vi "Update uService List.vi"(8 "error in (no error)":errorcluster, 10 "All uS?":bool, 11 "Common GUI v3 in":refnum<class "Common GUI v3.lvclass">) -> (0 "error out":errorcluster, 1 "Check currently displayed":set{string}(c389), 2 "For ComboBox":cluster{"ID":string, "ID":string}[](array[cluster]), 3 "Map":map{string, cluster{bool, "Last Pat":timestamp}}(c390), 5 "Common GUI v3 out":refnum<class "Common GUI v3.lvclass">)   [LabVIEW 2026, in "TALOS.lvlib" / "Common GUI v3.lvlib" / "Common GUI v3.lvclass"]
uses:
  Common GUI v3.lvclass
  Classes/uService List/uService List.lvclass/uService List.ctl
  Ancestor/Ancestor/Ancestor.lvclass/Ancestor.ctl
  Classes/uService List/Get all IDs.vi
  Classes/uService List/Get Properties.vi
  Support VIs/Generate Error.vi
  FGV/Error Memory/Get Error Description.vi
  Support VIs/Get PC name.vi
  Ancestor/Ancestor/Read ID.vi
  Support VIs/Get Class Name.vi
  <vilib>/Utility/error.llb/Clear Errors.vi
  FGV/Error Memory/Error Memory Core.vi
  <vilib>/AdvancedString/Delimited String to 1D String Array.vi
  <vilib>/AdvancedString/Delimited String to 1D String Array (string).vi
  Support VIs/Circus Root Path.vi
  FGV/Error Memory/Error Crt Lvl checker.vi
  FGV/Error Memory/Error Memory Core.vi/40c8088d-b597-4017-91af-faa98e00292e.vi
  FGV/Error Memory/Error Memory Core.vi/d4a3ab98-063c-4e44-b43d-fbdcfe6c2be2.vi
  Support VIs/Global Memory.vi
  <vilib>/Utility/LVClass/Get LV Class Name.vi
  Support VIs/Is in Packed Library.vi
  Support VIs/TALOS Root path.vi
  Support VIs/Read CSV worksheet.vi
  Support VIs/Global Constants.vi
  <vilib>/Utility/error.llb/General Error Handler.vi
  builds/Actor Framework PPL/Actor Framework.lvlibp/1abvi3w/vi.lib/ActorFramework/Message Enqueuer/Message Enqueuer.lvclass
  Ancestor/Ancestor/Ancestor.lvclass
  <vilib>/Comparison/Equal/Equal Functor/Equal Functor.lvclass
  Classes/uService List/uService List.lvclass
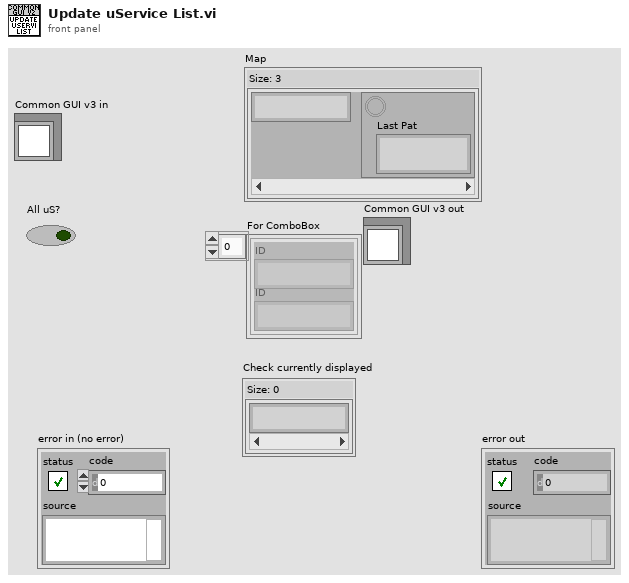
[diagram p1: front panel]
types:
  T1 = typedef "TALOS.lvlib/Classes.lvlib/uService List.lvclass/uService Properties.ctl" = cluster{"uService Queue":refnum<class "Message Enqueuer.lvclass">, "Last Pat":timestamp, "Online":bool, "Vi Ref":refnum<vi>, "Class name":string, "GUI":bool, "FP Items Refs Map":map{string, refnum<vi>}, "Remote GUI":bool, "Remote Window":refnum<vi>}
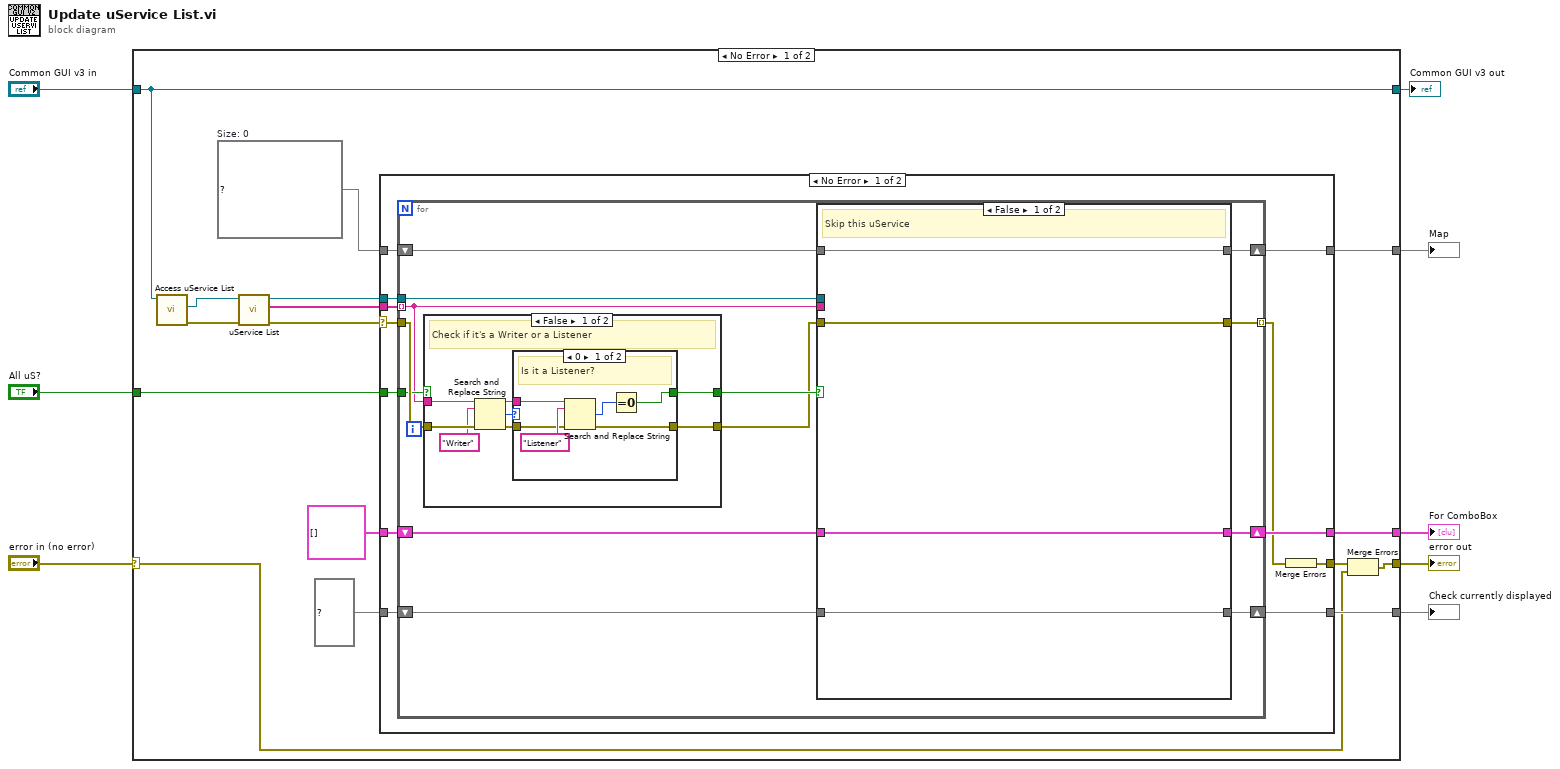
[diagram p0: block diagram]
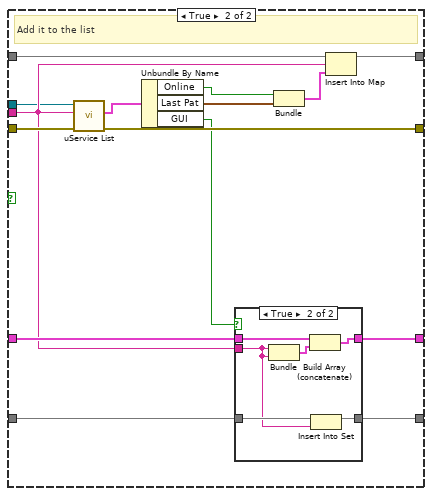
[diagram p2: hidden frame]
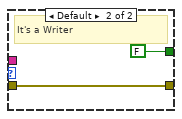
[diagram p4: hidden frame]
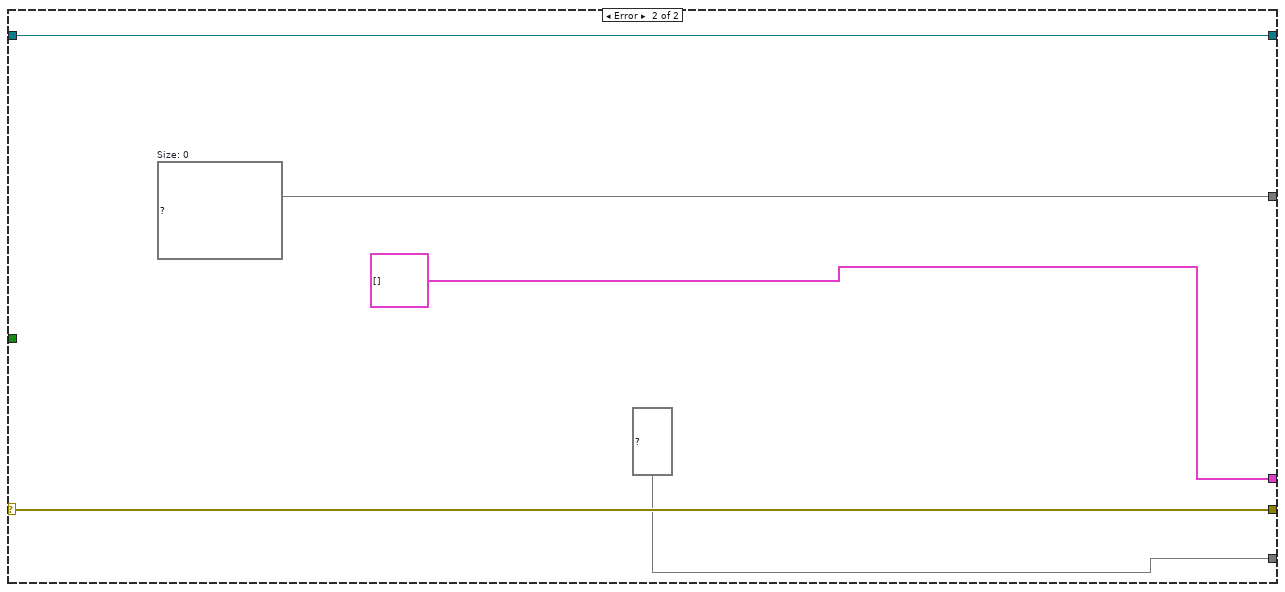
[diagram p7: hidden frame]
diagram:
  n1 = case shown="No Error" "error in (no error)" {
    selector: "error in (no error)" -> [w15 w103]
    tunnel: [w16 w103] -> w7
    tunnel: [w23 w102] -> w6
    tunnel: [w22 cluster{"ID":string, "ID":string}[] []] -> w5
    tunnel: [w17 set{string} {} ("Check currently displayed")] -> w4
    tunnel: "Common GUI v3 in" -> [w12 w99]
    tunnel: [w12 w99] -> w2
    tunnel: "All uS?" -> [w9 _]
    frame No Error {
      w24 = map{string, cluster{bool, "Last Pat":timestamp}} {}  # Size: 0
      n2 = call-dynamic "Access uService List.vi"("Ancestor in"=w12) -> ("error out"=w14:errorcluster, "uService List out"=w13:refnum<class "uService List.lvclass">)  [unwired: 8 in, 1 out]
      n3 = call-poly "uService List.vi"("error in (no error)"=w14, "uService List"=w13) -> ("error out"=w21:errorcluster, "All IDs"=w11:string[], "uService List out"=w10:refnum<class "uService List.lvclass">)  [unwired: 7 in]
      n4 = case shown="No Error" w21 {
        selector: w21 -> [w32 w95]
        tunnel: w24 -> [w36 w98]
        tunnel: [w35 w98] -> w23
        tunnel: [w34 w97] -> w22
        tunnel: w11 -> [w33 _]
        tunnel: cluster{"ID":string, "ID":string}[] [] -> [w31 w97]
        tunnel: [w29 w95] -> w19
        tunnel: set{string} {} ("Check currently displayed") -> [w28 w96]
        tunnel: [w27 w96] -> w17
        tunnel: w10 -> [w26 _]
        tunnel: w9 -> [w25 _]
        frame No Error {
          n5 = for {
            tunnel: w33 -> [w39] mode=indexing
            tunnel: w32 -> [w49]
            shift-right: [w48] -> w35
            shift-left: w36 -> [w47]
            shift-right: [w45] -> w34
            shift-left: w31 -> [w46]
            tunnel: [w44] -> w30 mode=indexing
            shift-right: [w42] -> w27
            shift-left: w28 -> [w43]
            tunnel: w26 -> [w41]
            tunnel: w25 -> [w40]
            n6 = case shown="False" w40 {
              selector: w40 -> [_ w94]
              tunnel: w39 -> [w84 _]
              tunnel: [w77 w94] -> w38
              tunnel: w49 -> [w83 w93]
              tunnel: [w78 w93] -> w37
              frame False {
                # "Check if it's a Writer or a Listener"
                n7 = Search and Replace String(input string=w84, search string="Writer", error in=w83) -> (result string=w79:string, number of replacements=w80:i32, error out=w81:errorcluster)  [unwired: 5 in, 1 out]
                n8 = case shown="0" w80 {
                  tunnel: w81 -> [w88 w92]
                  tunnel: w79 -> [w89 _]
                  tunnel: [w87 w92] -> w78
                  tunnel: [w85 FALSE] -> w77
                  frame 0 {
                    # "Is it a Listener?"
                    n9 = Search and Replace String(input string=w89, search string="Listener", error in=w88) -> (number of replacements=w86:i32, error out=w87:errorcluster)  [unwired: 5 in, 2 out]
                    n10 = Equal To 0?(x=w86) -> (x = 0?=w85:bool)
                  }
                  frame Default {
                    # "It's a Writer"
                  }
                }
              }
              frame True {
                # "Parse all uS"
              }
            }
            n11 = case shown="False" w38 {
              tunnel: [w53 w68] -> w48
              tunnel: w47 -> [w53 w67]
              tunnel: w46 -> [w51 w66]
              tunnel: [w51 w65] -> w45
              tunnel: w37 -> [w52 w64]
              tunnel: [w52 w63] -> w44
              tunnel: w43 -> [w50 w58]
              tunnel: [w50 w57] -> w42
              tunnel: w39 -> [_ w56]
              tunnel: w41 -> [_ w54]
              frame False {
                # "Skip this uService"
              }
              frame True {
                # "Add it to the list"
                n12 = call-poly "uService List.vi"("error in (no error)"=w64, "ID"=w56, "uService List in"=w54) -> ("error out"=w63:errorcluster, "uService Properties"=w55:T1)  [unwired: 6 in, 1 out]
                n13 = Unbundle By Name(w55) -> ("Online"=w60:bool, "Last Pat"=w61:timestamp, "GUI"=w62:bool)
                n14 = case shown="True" w62 {
                  tunnel: w66 -> [w70 w76]
                  tunnel: [w70 w74] -> w65
                  tunnel: w56 -> [_ w71]
                  tunnel: w58 -> [w69 w73]
                  tunnel: [w69 w72] -> w57
                  frame False {
                  }
                  frame True {
                    n15 = Bundle("ID"=w71, "ID"=w71) -> (w75:cluster{"ID":string, "ID":string})  [unwired: 1 in]
                    n16 = Build Array (concatenate)(w76, w75) -> (w74:cluster{"ID":string, "ID":string}[])
                    n17 = Insert Into Set(10:w71, 11:w73) -> (3:w72:set{string})  [unwired: 1 out]
                  }
                }
                n18 = Bundle("Online"=w60, "Last Pat"=w61) -> (w59:cluster{"Online":bool, "Last Pat":timestamp})  [unwired: 1 in]
                n19 = Insert Into Map(map in=w67, key=w56, value=w59) -> (map out=w68:map{string, cluster{bool, "Last Pat":timestamp}})  [unwired: 2 out]
              }
            }
          }
          n20 = Merge Errors(w30) -> (w29:errorcluster)
        }
        frame Error {
        }
      }
      n21 = Merge Errors(w19, w15) -> (w16:errorcluster)
    }
    frame Error {
      w102 = map{string, cluster{bool, "Last Pat":timestamp}} {}  # Size: 0
    }
  }
  "error out" <- w7
  "Map" <- w6
  "For ComboBox" <- w5
  "Check currently displayed" <- w4
  "Common GUI v3 out" <- w2
